vi "ADCP_Data_Packet_To_Raw_and_Processed_Bytes.vi"(0 "ADCP In":refnum<class "ADCP.lvclass">, 5 "Data Packet In":T2, 11 "error in (no error)":errorcluster) -> (4 "ADCP out":refnum<class "ADCP.lvclass">, 6 "Data Packet out":T2, 8 "Raw packet":u8[](array[numeric]), 10 "Processed packet":u8[](array[numeric]), 15 "error out":errorcluster)   [LabVIEW 2017, in "ADCP.lvclass"]
uses:
  ADCP.lvclass
  ADCP_Data_Packet_Transmit_Mode.ctl
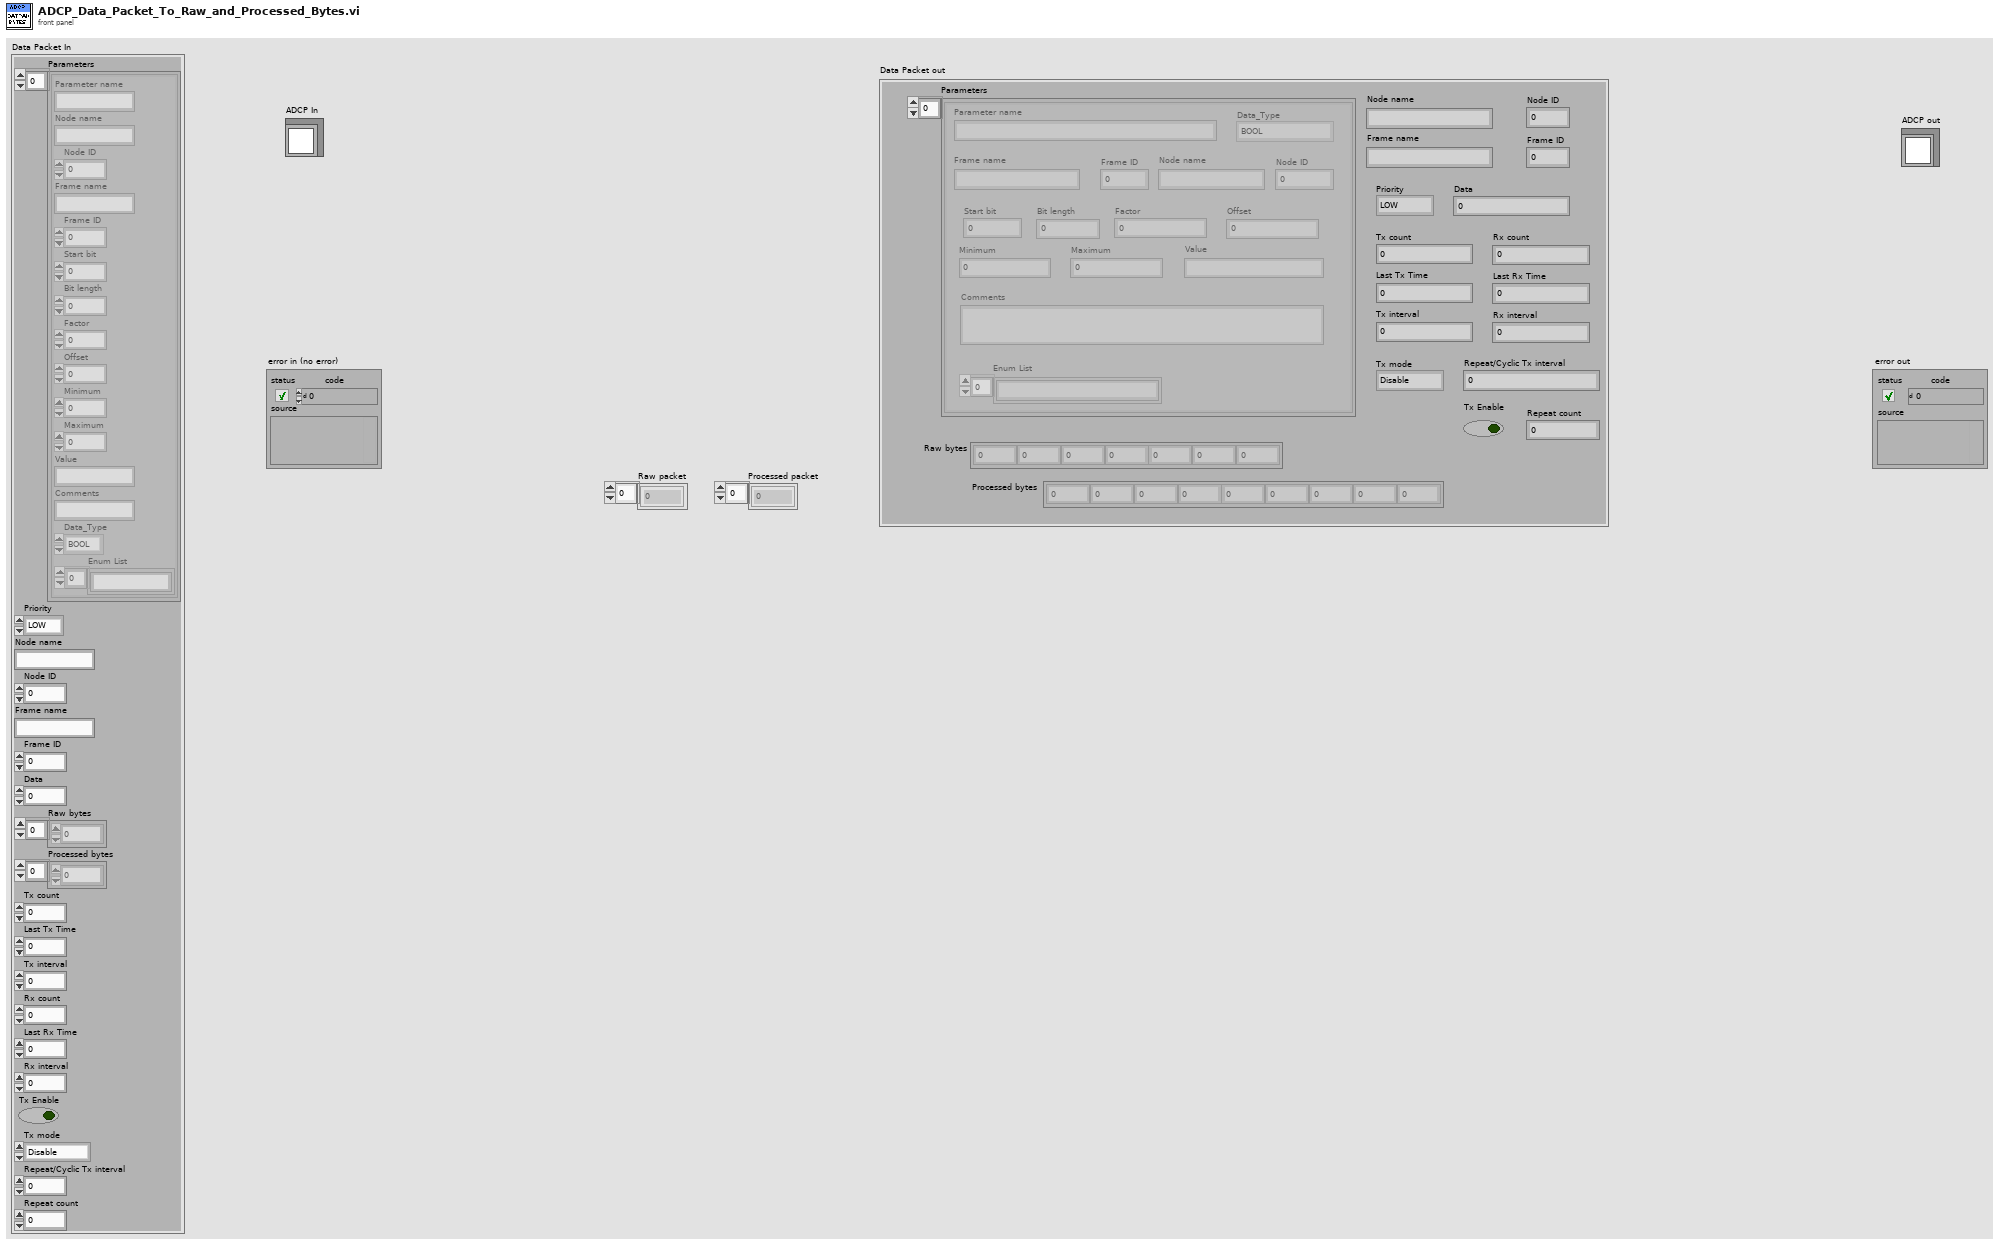
[diagram p1: front panel]
types:
  T1 = typedef "ADCP.lvclass/ADCP_Data_Packet_Transmit_Mode.ctl" = enum16{"Disable", "Single", "Cyclic", "Repeat"}
  T2 = cluster{"Parameters":cluster{"Parameter name":string, "Node name":string, "Node ID":u8, "Frame name":string, "Frame ID":u8, "Start bit":u32, "Bit length":u32, "Factor":dbl, "Offset":dbl, "Minimum":dbl, "Maximum":dbl, "Value":string, "Comments":string, "Data_Type":enum16{"BOOL", "UNSIGNED", "SIGNED", "FLOAT32", "ENUM"}, "Enum List":string[]}[], "Priority":enum16{"LOW", "HIGH"}, "Node name":string, "Node ID":u8, "Frame name":string, "Frame ID":u8, "Data":u32, "Raw bytes":u8[], "Processed bytes":u8[], "Tx count":i32, "Last Tx Time":u32, "Tx interval":u32, "Rx count":i32, "Last Rx Time":u32, "Rx interval":u32, "Tx Enable":bool, "Tx mode":T1, "Repeat/Cyclic Tx interval":u32, "Repeat count":u16}
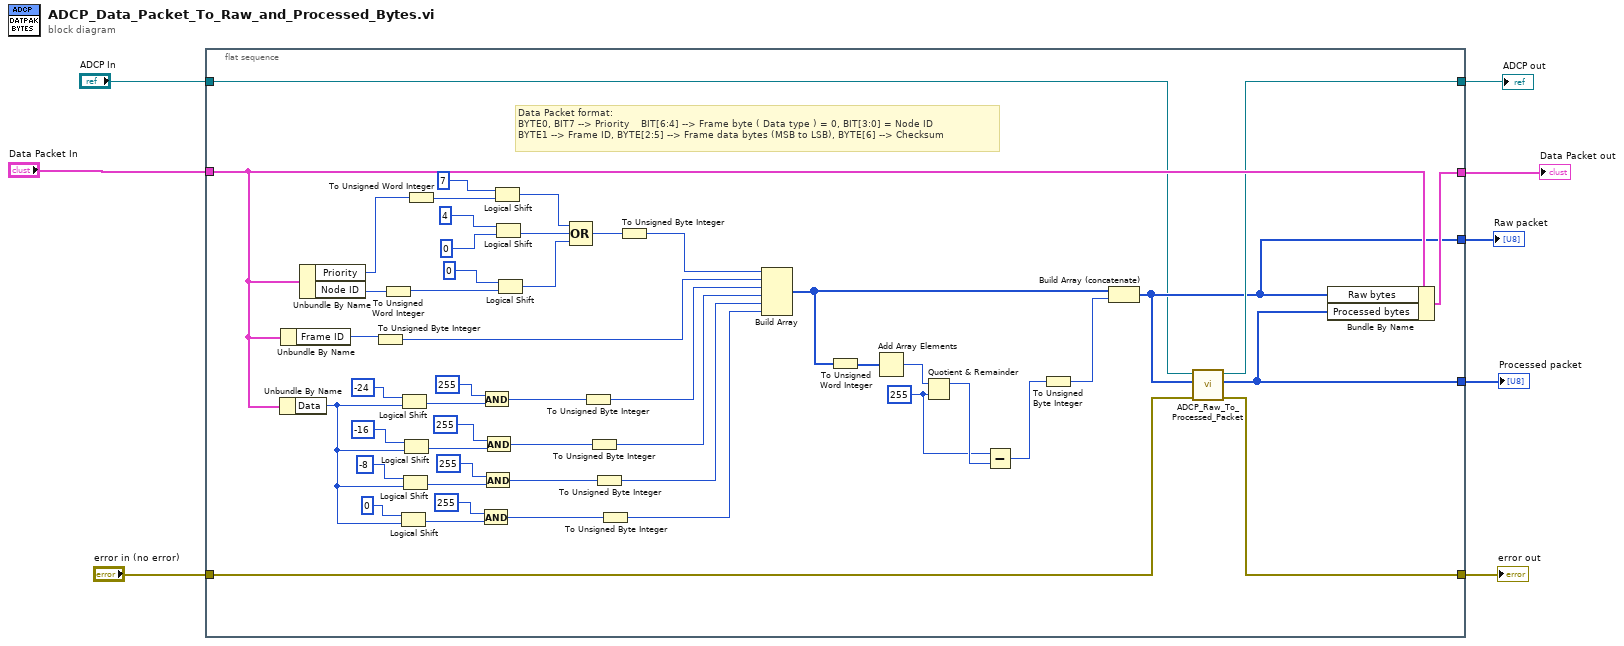
[diagram p0: block diagram]
diagram:
  n1 = flat-sequence {
    tunnel: "ADCP In" -> [w9]
    tunnel: "error in (no error)" -> [w16]
    tunnel: "Data Packet In" -> [w19]
    tunnel: [w17] -> w6
    tunnel: [w15] -> w5
    tunnel: [w18] -> w1
    tunnel: [w14] -> w4
    tunnel: [w13] -> w3
    frame #0 {
      w11 = u16 255 ("y")
      # "Data Packet format:\nBYTE0, BIT7 --> Priority    BIT[6:4] --> Frame byte ( Data type ) = 0, BIT[3:0] = Node ID\nBYTE1 --> Frame ID, BYTE[2:5] --> Frame data bytes (MSB to LSB), BYTE[6] --> Checksum"
      n2 = Unbundle By Name(w19) -> ("Data"=w32:u32)
      n3 = Unbundle By Name(w19) -> ("Frame ID"=w46:u8)
      n4 = Unbundle By Name(w19) -> ("Priority"=w59:enum16{"LOW", "HIGH"}, "Node ID"=w53:u8)
      n5 = To Unsigned Byte Integer(number=w46) -> (unsigned 8bit integer=w45:u8)
      n6 = To Unsigned Word Integer(number=w53) -> (unsigned 16bit integer=w52:u16)
      n7 = Logical Shift(y=i16 0, x=w32) -> (x << y=w34:u32)
      n8 = Logical Shift(y=i16 -24, x=w32) -> (x << y=w43:u32)
      n9 = Logical Shift(y=i16 -8, x=w32) -> (x << y=w37:u32)
      n10 = Logical Shift(y=i16 -16, x=w32) -> (x << y=w40:u32)
      n11 = To Unsigned Word Integer(number=w59) -> (unsigned 16bit integer=w58:u16)
      n12 = And(x=u32 255, y=w34) -> (x .and. y?=w26:u32)
      n13 = And(x=u32 255, y=w43) -> (x .and. y?=w31:u32)
      n14 = And(x=u32 255, y=w37) -> (x .and. y?=w27:u32)
      n15 = And(x=u32 255, y=w40) -> (x .and. y?=w29:u32)
      n16 = Logical Shift(y=i16 7, x=w58) -> (x << y=w51:u16)
      n17 = Logical Shift(y=i16 4, x=u16 0) -> (x << y=w50:u16)
      n18 = Logical Shift(y=i16 0, x=w52) -> (x << y=w49:u16)
      n19 = Compound Arithmetic op=OR(w51, w50, w49) -> (w48:u16)
      n20 = To Unsigned Byte Integer(number=w31) -> (unsigned 8bit integer=w30:u8)
      n21 = To Unsigned Byte Integer(number=w29) -> (unsigned 8bit integer=w28:u8)
      n22 = To Unsigned Byte Integer(number=w27) -> (unsigned 8bit integer=w25:u8)
      n23 = To Unsigned Byte Integer(number=w26) -> (unsigned 8bit integer=w24:u8)
      n24 = To Unsigned Byte Integer(number=w48) -> (unsigned 8bit integer=w47:u8)
      n25 = Build Array(w47, w45, w30, w28, w25, w24) -> (w21:u8[])
      n26 = To Unsigned Word Integer(number=w21) -> (unsigned 16bit integer=w23:u16[])
      n27 = Add Array Elements(numeric array=w23) -> (sum=w22:u16)
      n28 = Quotient & Remainder(x=w22, y=w11) -> (x-y*floor(x/y)=w12:u16)  [unwired: 1 out]
      n29 = Subtract(x=w11, y=w12) -> (x-y=w10:u16)
      n30 = To Unsigned Byte Integer(number=w10) -> (unsigned 8bit integer=w20:u8)
      n31 = Build Array (concatenate)(w21, w20) -> (w14:u8[])
      n32 = call "ADCP_Raw_To_Processed_Packet.vi"("error in (no error)"=w16, "Raw Packet"=w14, "ADCP in"=w9) -> ("error out"=w15:errorcluster, "Processed Packet"=w13:u8[], "ADCP out"=w17:refnum<class "ADCP.lvclass">)  [unwired: 6 in]
      n33 = Bundle By Name(cluster=w19, "Raw bytes"=w14, "Processed bytes"=w13) -> (w18:T2)
    }
  }
  "ADCP out" <- w6
  "error out" <- w5
  "Raw packet" <- w4
  "Processed packet" <- w3
  "Data Packet out" <- w1
